vi "Get AI Channel Count.vi"(3 "DAQ []":T1[](array[typedef]) {"AI.Coupling" items=["AC"=10045, "DC"=10050, "GND"=10066]}) -> (1 "# AI channels":i32)   [LabVIEW 2019, in "Instrument.Lockin.UI.lvclass"]
uses:
  Instrument.Lockin.UI.lvclass
  Typedefs/Device Configuration--Cluster.ctl
  Lockin.DAQ/Typedefs/446xAO-enum.ctl
  Lockin.DAQ/Typedefs/446xAI-enum.ctl
  Lockin.DAQ/Typedefs/AI.coupling-enum.ctl
  Instrument.Lockin/Instrument.Lockin.lvclass
  Lockin.DAQ/Lockin.DAQ.lvclass
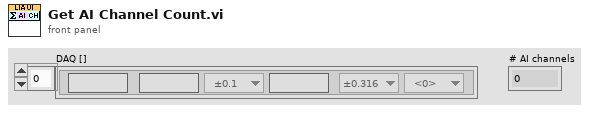
[diagram p1: front panel]
types:
  T1 = typedef "Instrument.Lockin.UI.lvclass/Device Configuration--Cluster.ctl" = cluster{"Device":string, "AO.Ch":string, "AO.Range":T2, "AI.Ch":string, "AI.Range":T3, "AI.Coupling":T4}
  T2 = typedef "Lockin.DAQ.lvclass/446xAO-enum.ctl" = enum16{"±0.1", "±1.0", "±10.0"}
  T3 = typedef "Lockin.DAQ.lvclass/446xAI-enum.ctl" = enum16{"±0.316", "±1.00", "±3.16", "±10.0", "±31.6", "±42.4"}
  T4 = typedef "Lockin.DAQ.lvclass/AI.coupling-enum.ctl" = u16
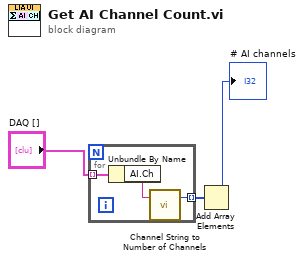
[diagram p0: block diagram]
diagram:
  n1 = for {
    tunnel: "DAQ []" -> [w6] mode=indexing
    tunnel: [w5] -> w1 mode=indexing
    n2 = Unbundle By Name(w6) -> ("AI.Ch"=w4:string)
    n3 = call "Channel String to Number of Channels.vi"("Channels String"=w4) -> ("# channels"=w5:i32)  [unwired: 2 in]
  }
  n4 = Add Array Elements(numeric array=w1) -> (sum=→"# AI channels":i32)
